vi "List Table.vi"(8 "error in (no error)":errorcluster, 11 "MySQL in":refnum<class "MySQL.lvclass">) -> (0 "error out":errorcluster, 2 "List Table":string[](array[string]), 3 "MySQL out":refnum<class "MySQL.lvclass">)   [LabVIEW 2021, in "Database.lvlib" / "MySQL.lvclass"]
uses:
  MySQL.lvclass
  DB/DB.lvclass
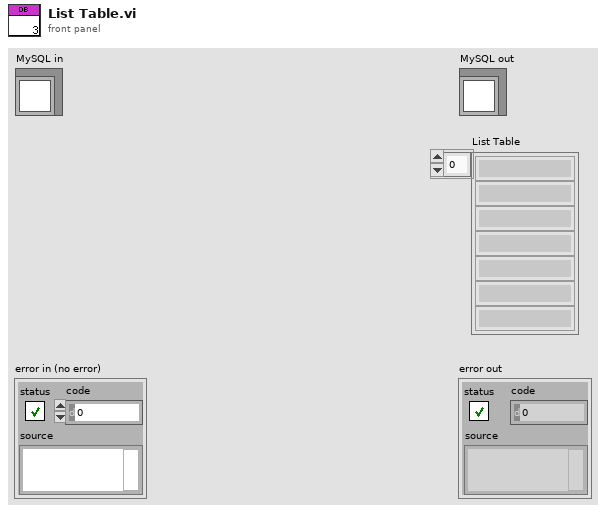
[diagram p1: front panel]
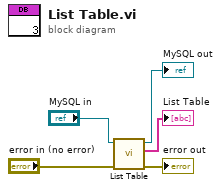
[diagram p0: block diagram]
diagram:
  n1 = call-parent "List Table.vi"("error in (no error)"="error in (no error)", "DB in"="MySQL in") -> ("error out"=→"error out":errorcluster, "List Table"=→"List Table":string[], "DB out"=→"MySQL out":refnum<class "MySQL.lvclass">)  [unwired: 7 in]
